vi "P1P2trig.vi"(10 "Phi2":bool, 11 "Phi1":bool) -> (1 "TrigUp":bool, 2 "Clock":bool, 3 "TrigDown":bool)   [LabVIEW 2012]
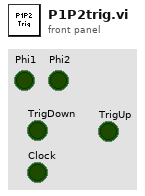
[diagram p1: front panel]
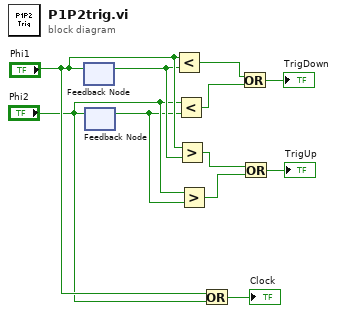
[diagram p0: block diagram]
diagram:
  n1 = feedback-in #1("Phi1") -> ()
  n2 = feedback #1() -> (w6:bool)  [unwired: 1 in]
  n3 = feedback #2() -> (w4:bool)  [unwired: 1 in]
  n4 = feedback-in #2("Phi2") -> ()
  n5 = Less?(x="Phi1", y=w6) -> (x < y?=w11:bool)
  n6 = Less?(x="Phi2", y=w4) -> (x < y?=w10:bool)
  n7 = Greater?(x="Phi1", y=w6) -> (0:w3:bool)
  n8 = Greater?(x="Phi2", y=w4) -> (0:w2:bool)
  n9 = Or(x="Phi1", y="Phi2") -> (x .or. y?=→"Clock":bool)
  n10 = Or(x=w11, y=w10) -> (x .or. y?=→"TrigDown":bool)
  n11 = Or(x=w3, y=w2) -> (x .or. y?=→"TrigUp":bool)
